vi "Create Channel Waveform.vi"(6 "Channel index":i32, 8 "error in (no error)":errorcluster, 10 "Data":i16[](array[numeric]), 11 "Pulse Driver in":refnum<class "Pulse Driver.lvclass">) -> (0 "error out":errorcluster, 1 "Waveform out":waveform(i16), 3 "Pulse Driver out":refnum<class "Pulse Driver.lvclass">)   [LabVIEW 2019, in "Pulse Driver.lvclass"]
uses:
  Pulse Driver.lvclass
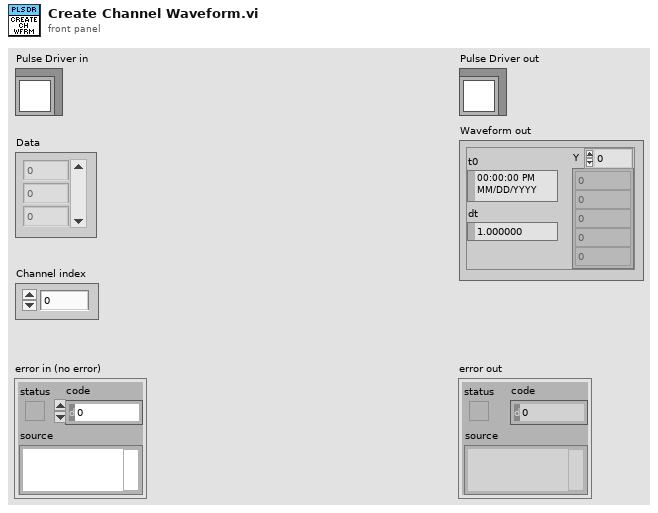
[diagram p1: front panel]
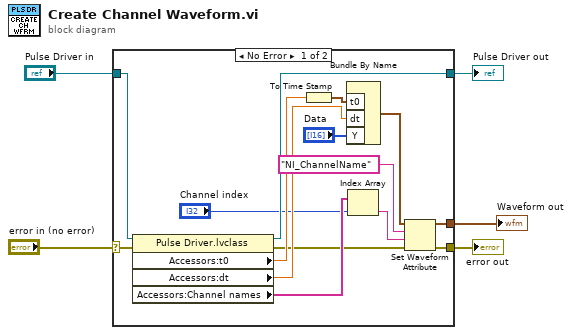
[diagram p0: block diagram]
diagram:
  n1 = case shown="No Error" "error in (no error)" {
    selector: "error in (no error)" -> [w8 w22]
    tunnel: [w7 w22] -> w4
    tunnel: [w19 w21] -> w2
    tunnel: "Pulse Driver in" -> [w20 w21]
    tunnel: [w6 _] -> w1
    frame No Error {
      n2 = property class="Pulse Driver.lvclass"(reference=w20, error in=w8) -> (reference out=w19:refnum<class "Pulse Driver.lvclass">, error out=w9:errorcluster, "Accessors:t0"=w18:dbl, "Accessors:dt"=w16:dbl, "Accessors:Channel names"=w13:string[])
      n3 = To Time Stamp(1:w18) -> (0:w17:timestamp)
      n4 = Bundle By Name("t0"=w17, "dt"=w16, "Y"="Data") -> (w14:waveform(i16))  [unwired: 1 out]
      n5 = Index Array(array=w13, index="Channel index") -> (element=w10:string)
      n6 = Set Waveform Attribute(4:w9, 5:w10, 6:"NI_ChannelName", 7:w14) -> (0:w7:errorcluster, 3:w6:waveform(i16))  [unwired: 1 out]
    }
    frame Error {
    }
  }
  "error out" <- w4
  "Pulse Driver out" <- w2
  "Waveform out" <- w1
